vi "CMN_Str2_2DArr.vi"(9 "col separator":string=",", 10 "multi line string in":string) -> (2 "array out":string[][](table))   [LabVIEW 2016]
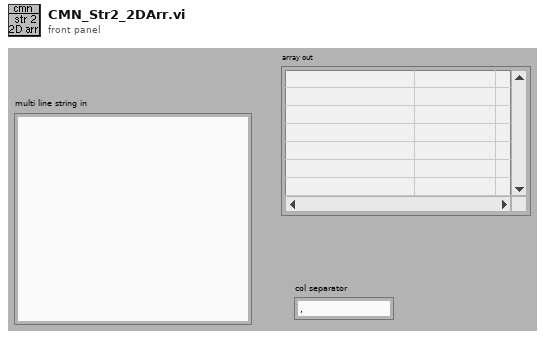
[diagram p1: front panel]
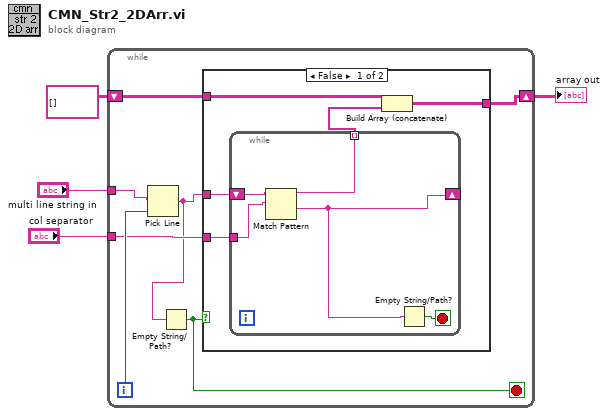
[diagram p0: block diagram]
diagram:
  n1 = while {
    tunnel: "col separator" -> [w10]
    tunnel: "multi line string in" -> [w5]
    shift-right: [w9] -> w1
    shift-left: string[][] [] -> [w8]
    i -> [w11]
    stop <- w6 stop-if-true
    n2 = Pick Line(multi-line string=w5, line index=w11) -> (output string=w7:string)  [unwired: 1 out]
    n3 = Empty String/Path?(string/path=w7) -> (empty?=w6:bool)
    n4 = case shown="False" w6 {
      tunnel: w7 -> [w16 _]
      tunnel: w10 -> [w15 _]
      tunnel: [w13 w22] -> w9
      tunnel: w8 -> [w12 w22]
      frame False {
        n5 = while {
          shift-right: [w18] -> _
          shift-left: w16 -> [w21]
          tunnel: w15 -> [w20]
          tunnel: [w17] -> w14 mode=indexing
          stop <- w19 stop-if-true
          n6 = Match Pattern(string=w21, regular expression=w20) -> (before substring=w17:string, after substring=w18:string)  [unwired: 3 out]
          n7 = Empty String/Path?(string/path=w18) -> (empty?=w19:bool)
        }
        n8 = Build Array (concatenate)(w12, w14) -> (w13:string[][])
      }
      frame True {
      }
    }
  }
  "array out" <- w1
